vi "test_gaussImageView.vi"() -> ()   [LabVIEW 2021]
panel:
  out "error out":errorcluster
  out "Intensity":sgl[][](array[numeric])
  in  "imageCols":i32=11
  in  "imageRows":i32=11
  in  "range":dbl=1.0
  in  "y pars":dbl[](array[numeric])=[1.0, 5.0, 3.0, 0.0]
  in  "x pars":dbl[](array[numeric])=[1.0, 5.0, 3.0, 0.0]
  out "Image viewer":T1(plugin-control)
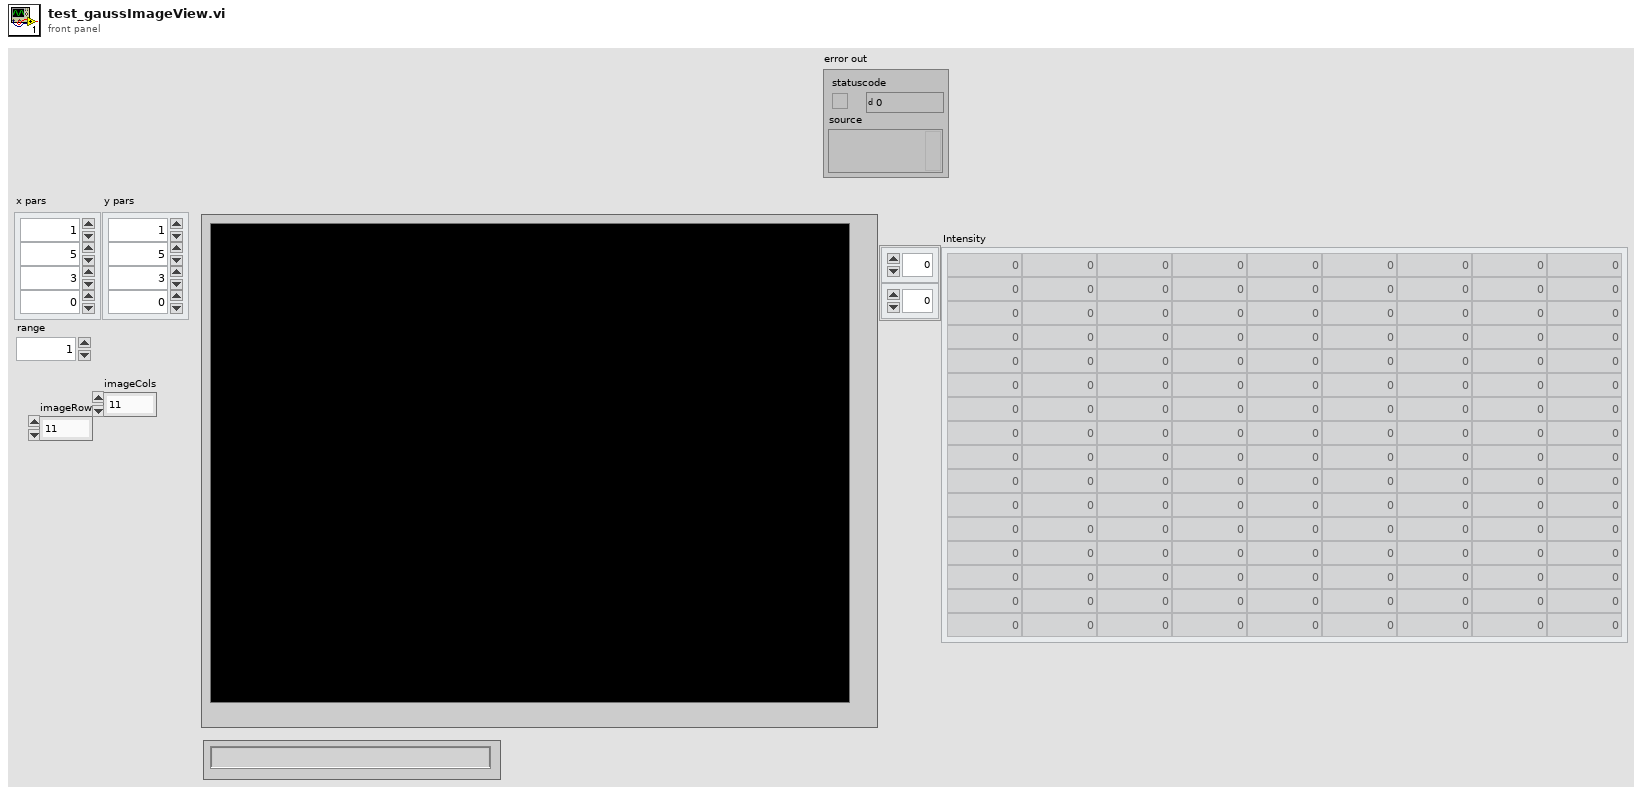
[diagram p1: front panel]
types:
  T1 = typedef "IMAQ Image.ctl" = refnum<image>
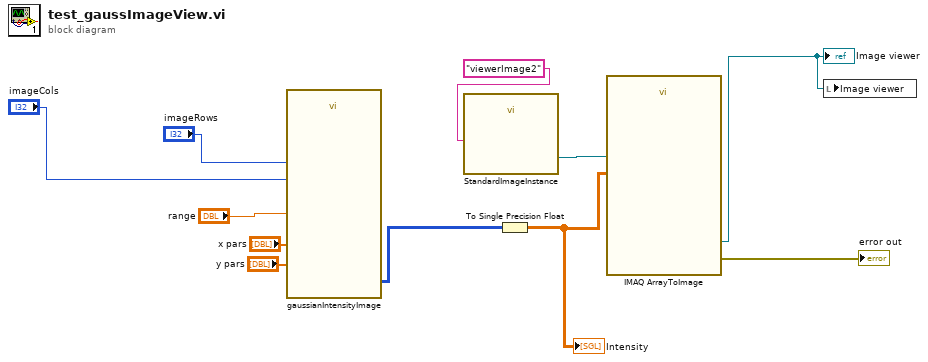
[diagram p0: block diagram]
diagram:
  n1 = call "gaussianIntensityImage.vi"("range"="range", "rows"="imageRows", "cols"="imageCols", "y pars"="y pars", "x pars"="x pars") -> ("Intesity"=w5:u32[][])  [unwired: 6 in]
  n2 = call "StandardImageInstance.vi"("Image Name"="viewerImage2") -> ("Refnum out"=w8:T1)  [unwired: 10 in]
  n3 = To Single Precision Float(number=w5) -> (single precision float=w4:sgl[][])
  "Intensity" <- w4
  n4 = call "IMAQ ArrayToImage"("Image Pixels (Float)"=w4, "Image"=w8) -> ("error out"=→"error out":errorcluster, "Image Out"=w9:T1)  [unwired: 8 in]
  "Image viewer" <- w9
  n5 = local write "Image viewer"(w9) -> ()
